vi "8-Axis (Manual) Coordinate Move.vi"() -> ()   [LabVIEW 2013]
uses:
  EMC API/EMC_Typedef_Motor_Parameters.ctl
  Typedef/Typedef_Motor_Action.ctl
  <vilib>/Motion/Express/_s/nimc.ex.power.power.axis.vi
  <vilib>/Motion/Express/_s/nimc.ex.resetPosition.resetPosition.axis.vi
  <vilib>/Motion/Express/_s/nimc.ex.findReferenceMove.startReferenceMove.axis.modeReverseLimit.vi
  <vilib>/Motion/Express/_s/nimc.ex.findReferenceMove.startReferenceMove.axis.modeHome.vi
  <vilib>/Motion/Express/_s/nimc.ex.findReferenceMove.startReferenceMove.axis.modeForwardLimit.vi
  <vilib>/Motion/Express/_s/nimc.ex.read.readTrajectoryData.axis.vi
  <vilib>/Motion/Express/_s/nimc.ex.read.readMotionIO.axis.vi
  <vilib>/Motion/BlockNode/FB.NIMotion.xnode
  Functional_Global/Typedef_FPGA_Interface_Action.ctl
  <vilib>/Motion/Express/_s/nimc.ex.clearFaults.clearFaults.axis.vi
panel:
  in  "resource":refnum<k21>="Axis 1"
  out "home active":bool
  out "rev. limit active":bool
  out "fwd. limit active":bool
  out "XY Graph":cluster{"X Array":dbl[], "Y Array":dbl[]}(graph)
  in  "interval":dbl=0.01 format="%#_13g"
  in  "Gear in/out":enum16{"Gear in", "Gear out"}(ring)
  in  "denominator":i32=1
  in  "numerator":i32=1
  in  "Master Axis":T1(ring)
  out "Array":dbl[](array[knob]) scale=0.0..1000.0
  in  "Clear Errors":bool
  in  "Command":T2
  in  "Motion Parameters":T3={"position"=1000.0, "velocity"=1000.0, "acceleration"=10000.0, "deceleration"=10000.0, "accel. jerk"=10000.0, "decel. jerk"=10000.0}
  in  "Axis Index":T1(ring)
  out "error":errorcluster
  out "Numeric":i32
  in  "Stop all motors":bool
  in  "Execute Command":bool
  in  "stop":bool
  out "Axis Velocities":T4(graph)
  out "Axis Positions":T4(graph)
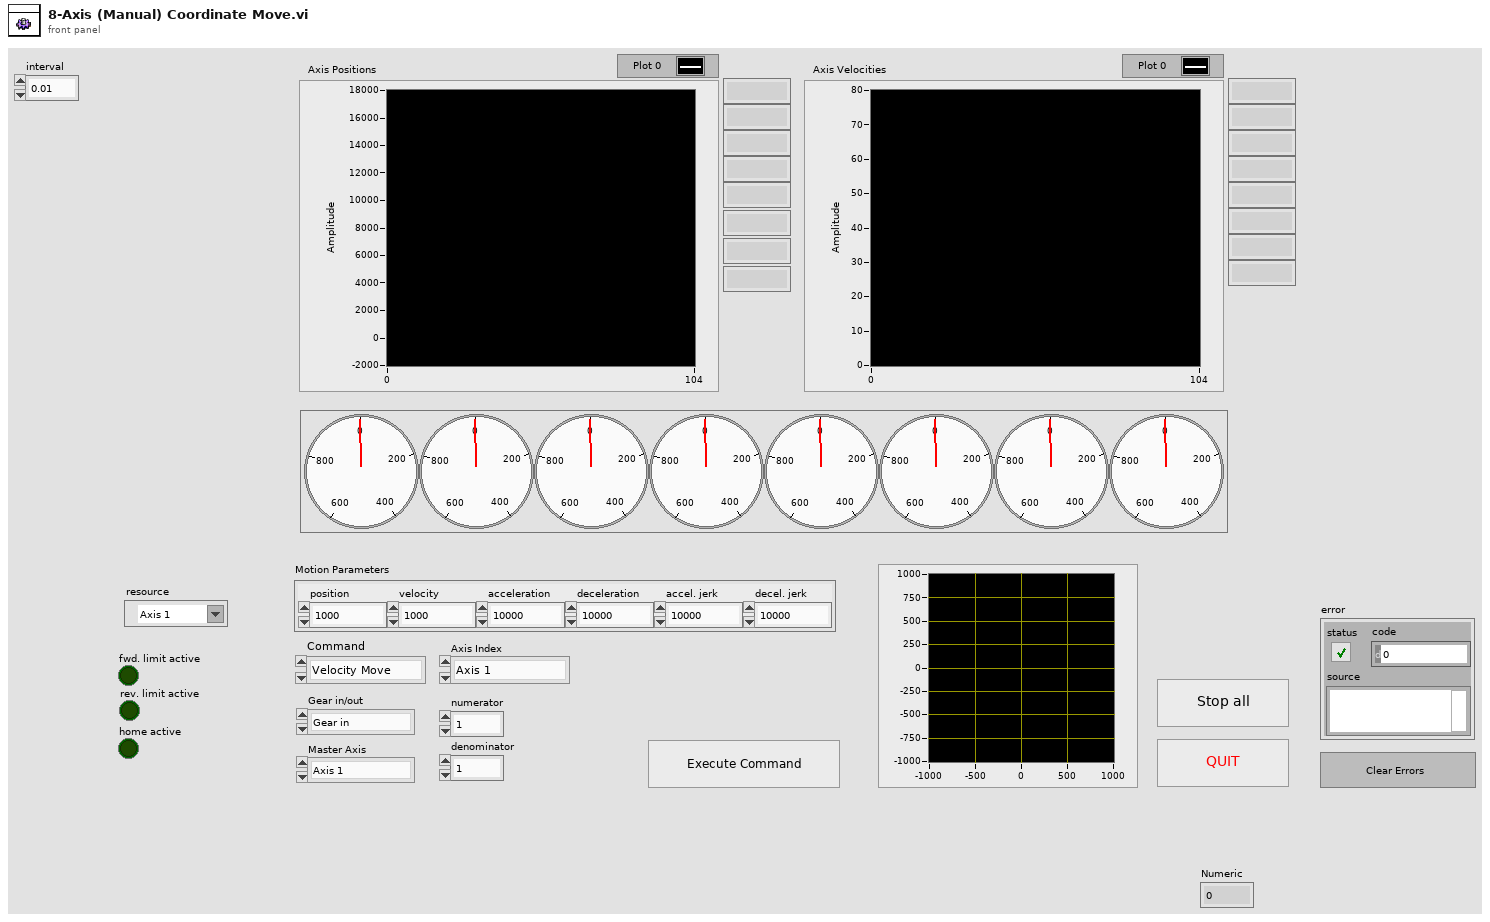
[diagram p1: front panel]
types:
  T1 = enum16{"Axis 1", "Axis 2", "Axis 3", "Axis 4", "Axis 5", "Axis 6", "Axis 7", "Axis 8"}
  T2 = typedef "Typedef_Motor_Action.ctl" = enum16{"Velocity Move", "REL Pos Move", "ABS Pos Move", "Stop", "Reset Position", "Contour_move", "Gearing", "Find Fwd Limit", "Find Rev Limit", "Find Home"}
  T3 = typedef "EMC_Typedef_Motor_Parameters.ctl" = cluster{"position":dbl, "velocity":dbl, "acceleration":dbl, "deceleration":dbl, "accel. jerk":dbl, "decel. jerk":dbl}
  T4 = cluster{"[0]":dbl, "[1]":dbl, "[2]":dbl, "[3]":dbl, "[4]":dbl, "[5]":dbl, "[6]":dbl, "[7]":dbl}
  T5 = typedef "Typedef_FPGA_Interface_Action.ctl" = enum16{"Initialize FPGA", "Get FPGA Reference", "Close FPGA"}
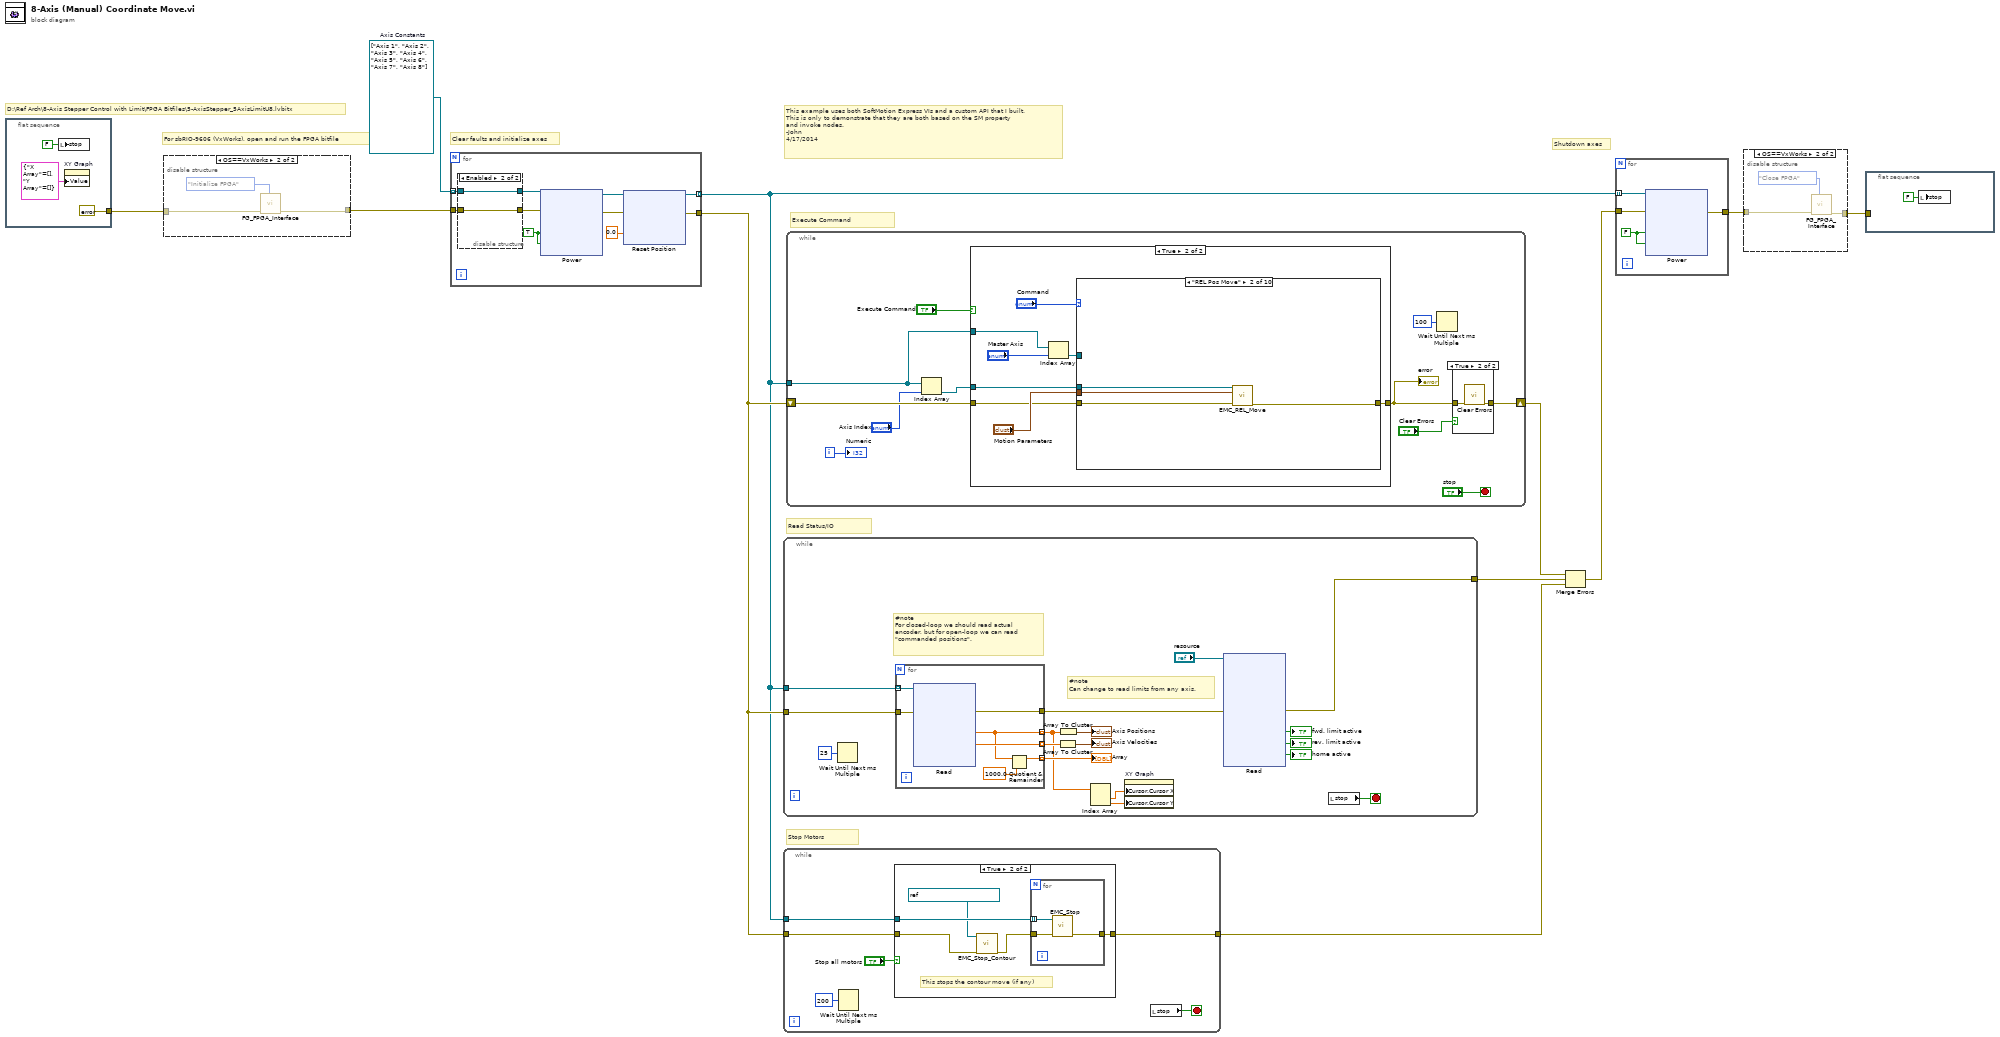
[diagram p0: block diagram]
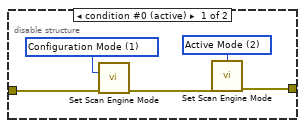
[diagram p3: hidden frame]
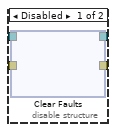
[diagram p4: hidden frame]
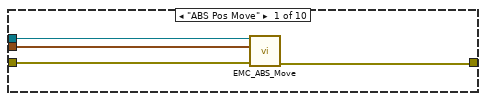
[diagram p8: hidden frame]
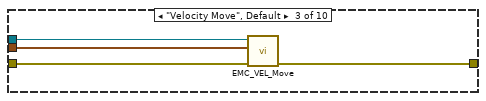
[diagram p9: hidden frame]
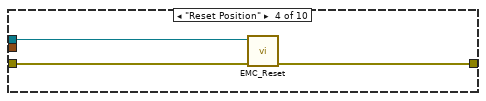
[diagram p10: hidden frame]
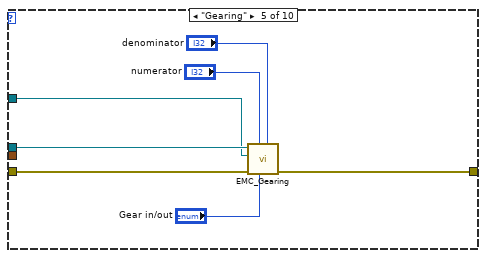
[diagram p11: hidden frame]
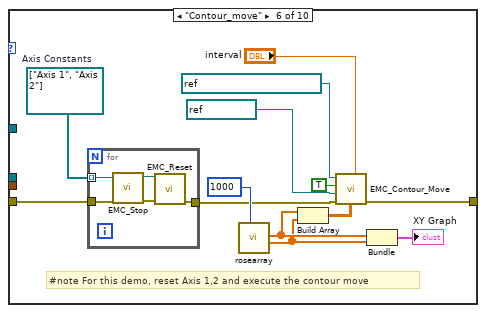
[diagram p12: hidden frame]
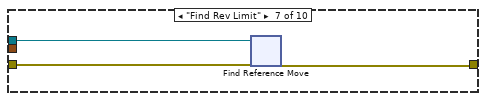
[diagram p13: hidden frame]
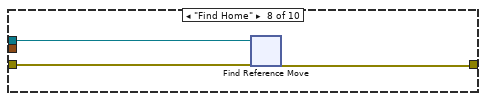
[diagram p14: hidden frame]
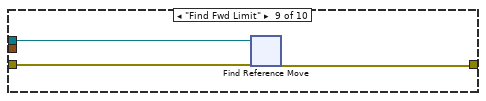
[diagram p15: hidden frame]
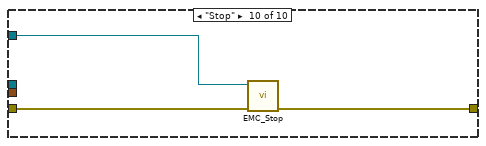
[diagram p16: hidden frame]
diagram:
  w10 = refnum<k21>[] ["Axis 1", "Axis 2", "Axis 3", "Axis 4", "Axis 5", "Axis 6", "Axis 7", "Axis 8"]  # Axis Constants
  # "For sbRIO-9606 (VxWorks), open and run the FPGA bitfile"
  # "D:\\Ref Arch\\8-Axis Stepper Control with Limit\\FPGA Bitfiles\\5-AxisStepper_5AxisLimitU8.lvbitx"
  # "Clear faults and initialize axes"
  # "This example uses both SoftMotion Express VIs and a custom API that I built.\nThis is only to demonstrate that they are both based on the SM property\nand invoke nodes. \n-John\n4/17/2014"
  # "Shutdown axes"
  # "Execute Command"
  # "Read Status/IO"
  # "Stop Motors"
  n1 = flat-sequence {
    tunnel: [errorcluster {"status"=FALSE, "code"=0, "source"=""} ("error in (no error)")] -> w7
    frame #0 {
      n2 = local write "stop"(FALSE ("stop")) -> ()
      n3 = property on="XY Graph" class="XYGraph (strict)"("Value"=cluster{"X Array":dbl[], "Y Array":dbl[]} {"X Array"=[], "Y Array"=[]} ("XY Graph")) -> ()  [unwired: 2 in, 2 out]
    }
  }
  n4 = disable-structure shown="OS==VxWorks" {
    disable-tunnel: [w19 w20] -> w3
    disable-tunnel: w7 -> [w18 w21]
    frame condition #0 (active) {
      w15 = 1 items=["Configuration Mode"=1, "Active Mode"=2] ("mode (Active Mode)")
      w16 = 2 items=["Configuration Mode"=1, "Active Mode"=2] ("mode (Active Mode)")
      n5 = call <vilib>:"Set Scan Engine Mode.vi"("mode (Active Mode)"=w15, "error in (no error)"=w18) -> ("error out"=w17:errorcluster)  [unwired: 13 in]
      n6 = call <vilib>:"Set Scan Engine Mode.vi"("mode (Active Mode)"=w16, "error in (no error)"=w17) -> ("error out"=w19:errorcluster)  [unwired: 13 in]
    }
    frame condition #1 {
      n7 = call "FG_FPGA_Interface.vi"("Action"=Typedef_FPGA_Interface_Action."Initialize FPGA", "error in"=w21) -> ("error out"=w20:errorcluster)  [unwired: 8 in, 1 out]
    }
  }
  n8 = for {
    tunnel: w10 -> [w26] mode=indexing
    tunnel: w3 -> [w25]
    tunnel: [w28] -> w2
    tunnel: [w27] -> w1 mode=indexing
    w32 = TRUE ("enable axis")
    n9 = disable-structure shown="Enabled" {
      disable-tunnel: w26 -> [w36 w42]
      disable-tunnel: w25 -> [w35 w41]
      disable-tunnel: [w34 w42] -> w24
      disable-tunnel: [w33 w41] -> w23
      frame Disabled {
        n10 = xnode ("Clear Faults")("resource"=w36, "error in"=w35) -> ("resource out"=w34:refnum<k21>, "error out"=w33:errorcluster)
      }
      frame Enabled {
      }
    }
    n11 = xnode ("Power")("enable axis"=w32, "enable drive"=w32, "resource"=w24, "error in"=w23) -> ("resource out"=w31:refnum<k21>, "error out"=w30:errorcluster)
    n12 = xnode ("Reset Position")("position"=0.0, "resource"=w31, "error in"=w30) -> ("resource out"=w27:refnum<k21>, "error out"=w28:errorcluster)
  }
  n13 = while {
    tunnel: w2 -> [w62]
    tunnel: w1 -> [w60]
    tunnel: [w58] -> w11
    stop <- w63 stop-if-true
    n14 = Wait Until Next ms Multiple(millisecond multiple=u32 200) -> ()  [unwired: 1 out]
    n15 = case shown="True" "Stop all motors" {
      tunnel: w62 -> [w64 w67]
      tunnel: [w64 w69] -> w58
      tunnel: w60 -> [_ w68]
      frame False {
      }
      frame True {
        # "This stops the contour move (if any)"
        n16 = call "EMC_Stop_Contour.vi"("error in (no error)"=w67, "coordinate"=refnum<k21> "Coordinate Space 1") -> ("error out"=w65:errorcluster)  [unwired: 9 in]
        n17 = for {
          tunnel: w65 -> [w72]
          tunnel: w68 -> [w70] mode=indexing
          tunnel: [w71] -> w69
          n18 = call "EMC_Stop.vi"("error in (no error)"=w72, "axis"=w70) -> ("error out"=w71:errorcluster)  [unwired: 8 in, 1 out]
        }
      }
    }
    n19 = local read "stop"() -> (w63:bool)
  }
  n20 = while {
    tunnel: w2 -> [w85]
    tunnel: w1 -> [w84]
    tunnel: [w73] -> w9
    stop <- w89 stop-if-true
    # "#note \nCan change to read limits from any axis."
    # "#note \nFor closed-loop we should read actual \nencoder, but for open-loop we can read\n\"commanded positions\"."
    n21 = Wait Until Next ms Multiple(millisecond multiple=u32 25) -> ()  [unwired: 1 out]
    n22 = for {
      tunnel: [w124] -> w75
      tunnel: [w119] -> w82 mode=indexing
      tunnel: [w123] -> w88 mode=indexing
      tunnel: w85 -> [w122]
      tunnel: w84 -> [w121] mode=indexing
      tunnel: [w118] -> w83 mode=indexing
      n23 = xnode ("Read")("resource"=w121, "error in"=w122) -> ("commanded position"=w119:dbl, "commanded vel."=w123:dbl, "error out"=w124:errorcluster)  [unwired: 2 out]
      n24 = Quotient & Remainder(x=w119, y=1000.0) -> (x-y*floor(x/y)=w118:dbl)  [unwired: 1 out]
    }
    "Array" <- w83
    n25 = Array To Cluster(array=w88) -> (cluster=→"Axis Velocities":T4)
    n26 = Array To Cluster(array=w82) -> (cluster=→"Axis Positions":T4)
    n27 = Index Array(array=w82) -> (element #1=w81:dbl, element #2=w80:dbl)  [unwired: 2 in]
    n28 = property on="XY Graph" class="XYGraph (strict)"("Cursor.Cursor X"=w81, "Cursor.Cursor Y"=w80) -> ()  [unwired: 2 in, 2 out]
    n29 = xnode ("Read")("resource"="resource", "error in"=w75) -> ("fwd. limit active"=→"fwd. limit active":bool, "rev. limit active"=→"rev. limit active":bool, "home active"=→"home active":bool, "error out"=w73:errorcluster)  [unwired: 6 out]
    n30 = local read "stop"() -> (w89:bool)
  }
  n31 = while {
    tunnel: w1 -> [w132]
    shift-right: [w133] -> w6
    shift-left: w2 -> [w137]
    i -> [w142]
    stop <- "stop" stop-if-true
    n32 = Index Array(array=w132, index="Axis Index") -> (element=w138:refnum<k21>)
    n33 = case shown="True" "Execute Command" {
      tunnel: w137 -> [w146 w153]
      tunnel: w138 -> [_ w152]
      tunnel: [w146 w151] -> w134
      tunnel: w132 -> [_ w148]
      frame False {
      }
      frame True {
        n34 = Index Array(array=w148, index="Master Axis") -> (element=w147:refnum<k21>)
        n35 = case shown="\"REL Pos Move\"" "Command" {
          tunnel: "Motion Parameters" -> [w155 w159 w166 _ _ _ _ _ _ _]
          tunnel: w153 -> [w158 w162 w165 w169 w176 w179 w196 w215 w236 w256]
          tunnel: w152 -> [w156 w160 w164 w168 w175 _ w195 w214 w235 _]
          tunnel: [w157 w161 w163 w167 w174 w189 w197 w216 w237 w255] -> w151
          tunnel: w147 -> [_ _ _ _ w170 _ _ _ _ w254]
          frame "ABS Pos Move" {
            n36 = call "EMC_ABS_Move.vi"("error in (no error)"=w158, "Motion Parameters"=w155, "axis"=w156) -> ("error out"=w157:errorcluster)  [unwired: 8 in]
          }
          frame "REL Pos Move" {
            n37 = call "EMC_REL_Move.vi"("error in (no error)"=w162, "Motion Parameters"=w159, "axis"=w160) -> ("error out"=w161:errorcluster)  [unwired: 8 in]
          }
          frame "Velocity Move", Default {
            n38 = call "EMC_VEL_Move.vi"("error in (no error)"=w165, "Motion Parameters"=w166, "axis"=w164) -> ("error out"=w163:errorcluster)  [unwired: 8 in]
          }
          frame "Reset Position" {
            n39 = call "EMC_Reset.vi"("error in (no error)"=w169, "axis"=w168) -> ("error out"=w167:errorcluster)  [unwired: 9 in]
          }
          frame "Gearing" {
            n40 = call "EMC_Gearing.vi"("denominator"="denominator", "Gear in/out"="Gear in/out", "numerator"="numerator", "error in (no error)"=w176, "master axis"=w170, "axis"=w175) -> ("error out"=w174:errorcluster)  [unwired: 5 in]
          }
          frame "Contour_move" {
            w177 = refnum<k21>[] ["Axis 1", "Axis 2"]  # Axis Constants
            # "#note For this demo, reset Axis 1,2 and execute the contour move"
            n41 = for {
              tunnel: w179 -> [w193]
              tunnel: [w194] -> w178
              tunnel: w177 -> [w191] mode=indexing
              n42 = call "EMC_Stop.vi"("error in (no error)"=w193, "axis"=w191) -> ("error out"=w192:errorcluster, "axis out"=w190:refnum<k21>)  [unwired: 8 in]
              n43 = call "EMC_Reset.vi"("error in (no error)"=w192, "axis"=w190) -> ("error out"=w194:errorcluster)  [unwired: 9 in]
            }
            n44 = call "rosearray.vi"("Iterations"=u32 1000) -> ("Y Array"=w181:dbl[], "X Array"=w182:dbl[])  [unwired: 5 in, 1 out]
            n45 = Build Array(w182, w181) -> (w185:dbl[][])
            n46 = call "EMC_Contour_Move.vi"("interval"="interval", "points[][]"=w185, "error in (no error)"=w178, "table"=refnum<k21> "Table 1" ("resource"), "overwrite"=TRUE, "coordinate"=refnum<k21> "Coordinate Space 1" ("resource")) -> ("error out"=w189:errorcluster)  [unwired: 5 in]
            n47 = Bundle("X Array"=w182, "Y Array"=w181) -> (→"XY Graph":cluster{"X Array":dbl[], "Y Array":dbl[]})  [unwired: 1 in]
          }
          frame "Find Rev Limit" {
            n48 = xnode "Find Reference Move"("resource"=w195, "error in"=w196) -> ("error out"=w197:errorcluster)  [unwired: 9 in, 2 out]
          }
          frame "Find Home" {
            n49 = xnode "Find Reference Move"("resource"=w214, "error in"=w215) -> ("error out"=w216:errorcluster)  [unwired: 11 in, 2 out]
          }
          frame "Find Fwd Limit" {
            n50 = xnode "Find Reference Move"("resource"=w235, "error in"=w236) -> ("error out"=w237:errorcluster)  [unwired: 9 in, 2 out]
          }
          frame "Stop" {
            n51 = call "EMC_Stop.vi"("error in (no error)"=w256, "axis"=w254) -> ("error out"=w255:errorcluster)  [unwired: 8 in, 1 out]
          }
        }
      }
    }
    "error" <- w134
    n52 = Wait Until Next ms Multiple(millisecond multiple=u32 100) -> ()  [unwired: 1 out]
    n53 = case shown="True" "Clear Errors" {
      tunnel: w134 -> [w143 w145]
      tunnel: [w143 w144] -> w133
      frame False {
      }
      frame True {
        n54 = call <vilib>:"Clear Errors.vi"("error in (no error)"=w145) -> ("error out"=w144:errorcluster)  [unwired: 6 in]
      }
    }
    "Numeric" <- w142
  }
  n55 = Merge Errors(w6, w9, w11) -> (w5:errorcluster)
  n56 = for {
    tunnel: w1 -> [w260] mode=indexing
    tunnel: [w258] -> w4
    tunnel: w5 -> [w257]
    w259 = FALSE ("enable axis")
    n57 = xnode ("Power")("enable axis"=w259, "enable drive"=w259, "resource"=w260, "error in"=w257) -> ("error out"=w258:errorcluster)  [unwired: 1 out]
  }
  n58 = disable-structure shown="OS==VxWorks" {
    disable-tunnel: w4 -> [w271 w273]
    disable-tunnel: [w271 w272] -> w8
    frame condition #0 (active) {
    }
    frame condition #1 {
      n59 = call "FG_FPGA_Interface.vi"("Action"=Typedef_FPGA_Interface_Action."Close FPGA", "error in"=w273) -> ("error out"=w272:errorcluster)  [unwired: 8 in, 1 out]
    }
  }
  n60 = flat-sequence {
    tunnel: w8 -> [_]
    frame #0 {
      n61 = local write "stop"(FALSE ("stop")) -> ()
    }
  }
